vi "Set Message Name.vi"(8 "error in":errorcluster, 10 "name":string, 11 "message or subaddress":T1 format="%.0x") -> (0 "error out":errorcluster, 3 "message or subaddress out":T1 format="%.0x")   [LabVIEW 2020, in "AIM MIL-STD-1553 Scripting.lvlib"]
doc: "Sets the <b>name</b> of the input <b>message or subaddress</b>."
uses:
  AIM MIL-STD-1553 Scripting.lvlib
  <vilib>/NI VeriStand/Custom Device API/Custom Device Item Ref.ctl
  Constants.vi
  <vilib>/NI VeriStand/Custom Device API/Set Item Property (String).vi
  <vilib>/NI VeriStand/Custom Device API/Custom Device API.lvlib
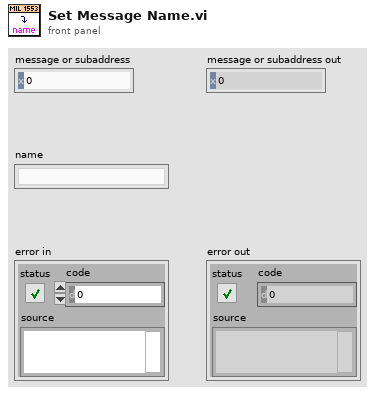
[diagram p1: front panel]
types:
  T1 = typedef "Custom Device API.lvlib/Custom Device Item Ref.ctl" = u64
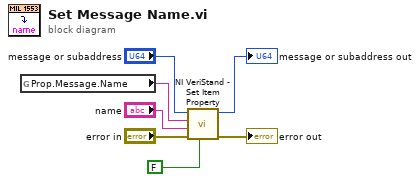
[diagram p0: block diagram]
diagram:
  n1 = global read "Constants.vi" "Prop.Message.Name"() -> (w3:string)
  n2 = call-poly <vilib>:"NI VeriStand - Set Item Property.vi"("Binary String (T)"=FALSE, "error in (no error)"="error in", "Value"="name", "Property Name"=w3, "Item Ref in"="message or subaddress") -> ("error out"=→"error out":errorcluster, "Item Ref out"=→"message or subaddress out":T1)  [unwired: 4 in, 1 out]
